vi "Plant Simulator.vi"(0 "Initial PV":dbl format="%.2f", 1 "dt (s)":dbl=-1.0 format="%.3f", 2 "Measurement Noise (%)":dbl(slide) scale=0.0..100.0, 4 "Controller Noise (%)":dbl(slide) scale=0.0..100.0, 5 "Valve Deadband":dbl format="%.1f", 6 "Process Deadtime":i32(slide) scale=0.0..5.0, 7 "Lag (min)":dbl format="%.2f", 8 "Process Load":dbl(slide) scale=0.0..50.0, 9 "Process Gain":dbl(slide)=1.0 scale=0.0..5.0, 10 "Manipulated Variable (Output, %)":dbl format="%.2f", 11 "Reinitialize":bool) -> (3 "Process Variable (%)":dbl format="%.2f")   [LabVIEW 2023]
doc: "Simulates a physical plant's response; for use with feedback control loops.\n\nAll scale factors are in percent. Lag time is in minutes. Process Deadtime is a true deadtime, measured as a multiple of the loop cycle time. NOTE: this deadtime is dependent upon the interval at which this VI is called. You can modify the algorithm used here to simulate almost any process.\n\nIf more than one plant needs to be simulated simultaneously, save multiple copies of this VI under different names."
uses:
  <vilib>/addons/control/pid/pid.llb/PID Lead-Lag (DBL).vi
  <vilib>/addons/control/pid/NI_PID_pid.lvlib
panel:
  # "Plant Characteristics"
  # "(x cycle time)"
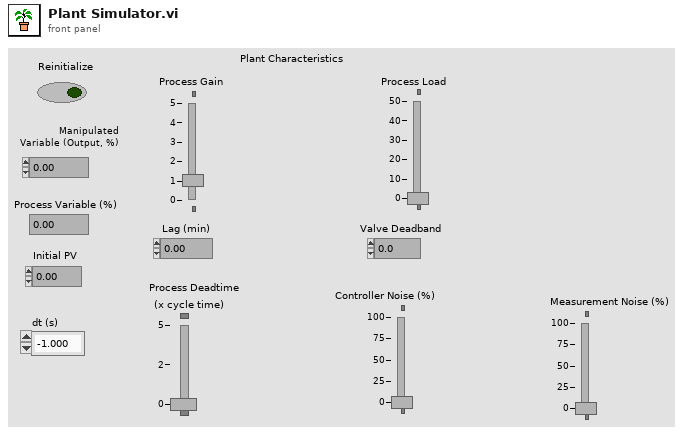
[diagram p1: front panel]
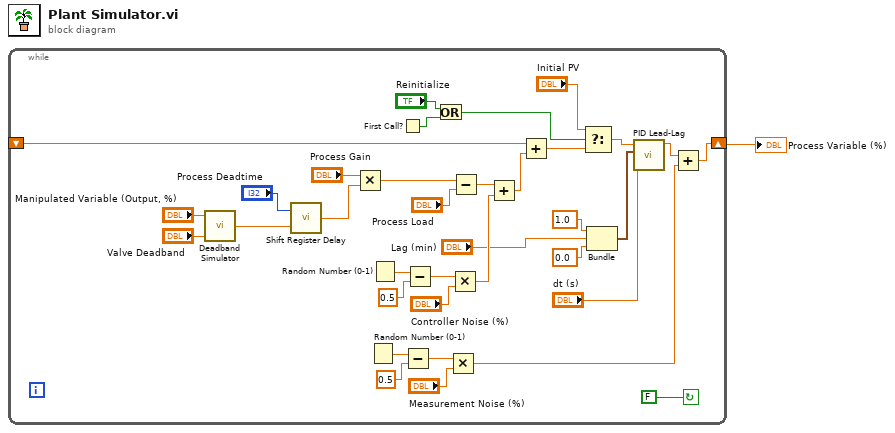
[diagram p0: block diagram]
diagram:
  n1 = while {
    shift-left: _ -> [w13]
    shift-right: [w6] -> w1
    stop <- FALSE continue-if-true
    n2 = call "Deadband Simulator.vi"("deadband (%)"="Valve Deadband", "requested pos. (%)"="Manipulated Variable (Output, %)") -> ("actual pos. (%)"=w36:dbl)  [unwired: 1 in]
    n3 = call "Shift Register Delay.vi"("input"=w36, "n delay (0)"="Process Deadtime") -> ("output"=w32:dbl)
    n4 = Multiply(x="Process Gain", y=w32) -> (x*y=w23:dbl)
    n5 = Random Number (0-1)() -> (number: 0 to 1=w11:dbl)
    n6 = Random Number (0-1)() -> (number: 0 to 1=w22:dbl)
    n7 = First Call?() -> (First Call?: T/F=w2:bool)
    n8 = Subtract(x=w11, y=0.5) -> (x-y=w9:dbl)
    n9 = Subtract(x=w22, y=0.5) -> (x-y=w29:dbl)
    n10 = Or(x="Reinitialize", y=w2) -> (x .or. y?=w3:bool)
    n11 = Multiply(x=w9, y="Measurement Noise (%)") -> (x*y=w5:dbl)
    n12 = Multiply(x=w29, y="Controller Noise (%)") -> (x*y=w35:dbl)
    n13 = Subtract(x=w23, y="Process Load") -> (x-y=w24:dbl)
    n14 = Add(x=w24, y=w35) -> (x+y=w28:dbl)
    n15 = Add(x=w13, y=w28) -> (x+y=w18:dbl)
    n16 = Select(t="Initial PV", s=w3, f=w18) -> (s? t:f=w17:dbl)
    n17 = Bundle(1.0, "Lag (min)"="Lag (min)", 0.0) -> (w14:cluster{dbl, "Lag (min)":dbl, dbl})  [unwired: 1 in]
    n18 = call-poly <vilib>:"PID Lead-Lag.vi"("dt (s)"="dt (s)", "tuning parameters"=w14, "input"=w17) -> ("output"=w7:dbl)  [unwired: 5 in, 1 out]
    n19 = Add(x=w7, y=w5) -> (x+y=w6:dbl)
  }
  "Process Variable (%)" <- w1
